vi "Com _Circuit Compare.vi"(8 "error in (no error)":errorcluster caption="错误输入（无错误）", 9 "tblName":string, 10 "PCBANo":string, 11 "Traceability 引用句柄":refnum<k24>) -> (0 "error out":errorcluster caption="错误输出", 2 ".NET:System.Data.DataSet":T1={"CaseSensitive"=FALSE, "Container"=refnum, "DataSetName"="", "DefaultViewManager"=refnum, "DesignMode"=FALSE, "EnforceConstraints"=FALSE, "ExtendedProperties"=refnum, "HasErrors"=FALSE, "IsInitialized"=FALSE, "Locale"=refnum, "Namespace"="", "Prefix"="", "Relations"=refnum, "RemotingFormat"=0, "SchemaSerializationMode"=1, "Site"=refnum, "Tables"=refnum} {"SchemaSerializationMode" items=["IncludeSchema"=1, "ExcludeSchema"=2]; "RemotingFormat" items=["Xml", "Binary"]}, 3 "Traceability 引用句柄输出":refnum<k24>)   [LabVIEW 2014, in "Traceability.lvlib"]
uses:
  D:/webservice/Traceability.dll
  Traceability.dll
  System.Data
  Traceability.lvlib
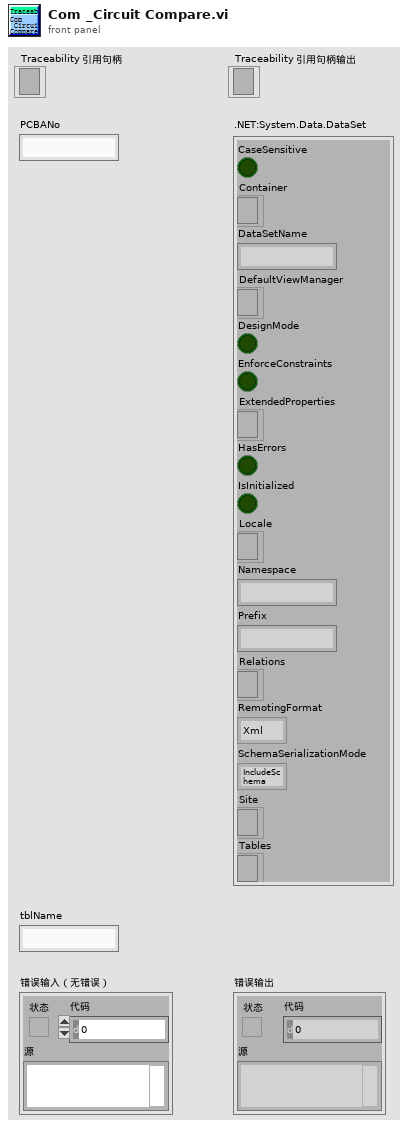
[diagram p1: front panel]
types:
  T1 = cluster{"CaseSensitive":bool, "Container":refnum<k24>, "DataSetName":string, "DefaultViewManager":refnum<k24>, "DesignMode":bool, "EnforceConstraints":bool, "ExtendedProperties":refnum<k24>, "HasErrors":bool, "IsInitialized":bool, "Locale":refnum<k24>, "Namespace":string, "Prefix":string, "Relations":refnum<k24>, "RemotingFormat":i32, "SchemaSerializationMode":i32, "Site":refnum<k24>, "Tables":refnum<k24>}
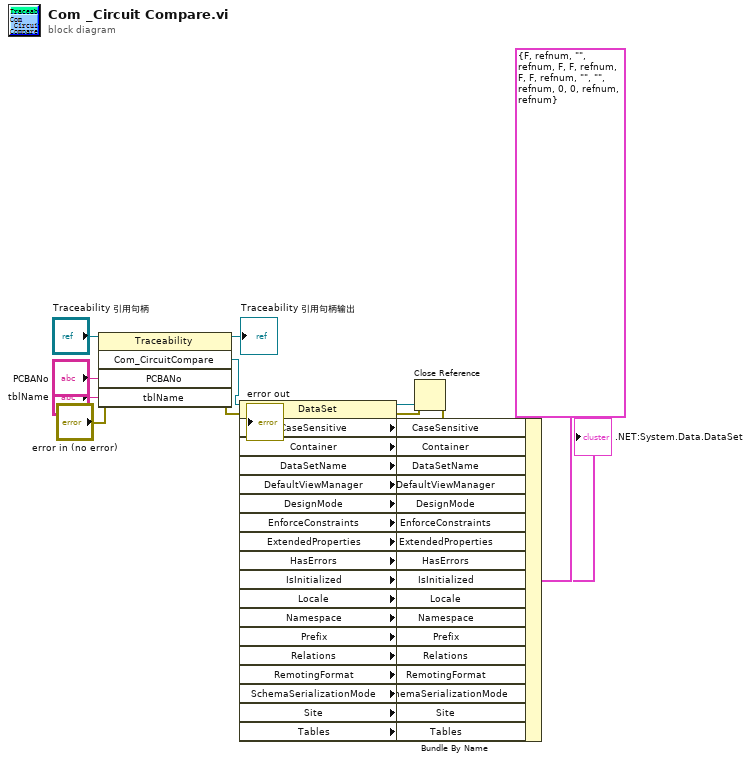
[diagram p0: block diagram]
diagram:
  n1 = invoke class="Traceability" method="Com_CircuitCompare"(reference="Traceability 引用句柄", error in="error in (no error)", "PCBANo"="PCBANo", "tblName"="tblName") -> (reference out=→"Traceability 引用句柄输出":refnum<k24>, error out=w4:errorcluster, "Com_CircuitCompare"=w26:refnum<k24>)  [unwired: 1 in, 2 out]
  n2 = property class="DataSet"(reference=w26, error in=w4) -> (reference out=w3:refnum<k24>, error out=w2:errorcluster, "CaseSensitive"=w23:bool, "Container"=w22:refnum<k24>, "DataSetName"=w21:string, "DefaultViewManager"=w20:refnum<k24>, "DesignMode"=w19:bool, "EnforceConstraints"=w18:bool, "ExtendedProperties"=w17:refnum<k24>, "HasErrors"=w16:bool, "IsInitialized"=w15:bool, "Locale"=w14:refnum<k24>, "Namespace"=w13:string, "Prefix"=w12:string, "Relations"=w11:refnum<k24>, "RemotingFormat"=w10:i32, "SchemaSerializationMode"=w9:i32, "Site"=w8:refnum<k24>, "Tables"=w7:refnum<k24>)
  n3 = Bundle By Name(cluster=T1 {"CaseSensitive"=FALSE, "Container"=refnum, "DataSetName"="", "DefaultViewManager"=refnum, "DesignMode"=FALSE, "EnforceConstraints"=FALSE, "ExtendedProperties"=refnum, "HasErrors"=FALSE, "IsInitialized"=FALSE, "Locale"=refnum, "Namespace"="", "Prefix"="", "Relations"=refnum, "RemotingFormat"=0, "SchemaSerializationMode"=0, "Site"=refnum, "Tables"=refnum} (".NET:System.Data.DataSet"), "CaseSensitive"=w23, "Container"=w22, "DataSetName"=w21, "DefaultViewManager"=w20, "DesignMode"=w19, "EnforceConstraints"=w18, "ExtendedProperties"=w17, "HasErrors"=w16, "IsInitialized"=w15, "Locale"=w14, "Namespace"=w13, "Prefix"=w12, "Relations"=w11, "RemotingFormat"=w10, "SchemaSerializationMode"=w9, "Site"=w8, "Tables"=w7) -> (→".NET:System.Data.DataSet":T1)
  n4 = Close Reference(reference=w3, error in (no error)=w2) -> (error out=→"error out":errorcluster)
